vi "Load Words.vi"() -> (3 "Words":string[](array[string]))   [LabVIEW 2020]
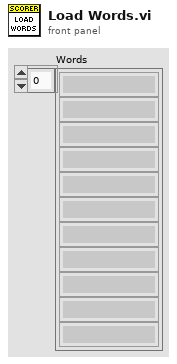
[diagram p1: front panel]
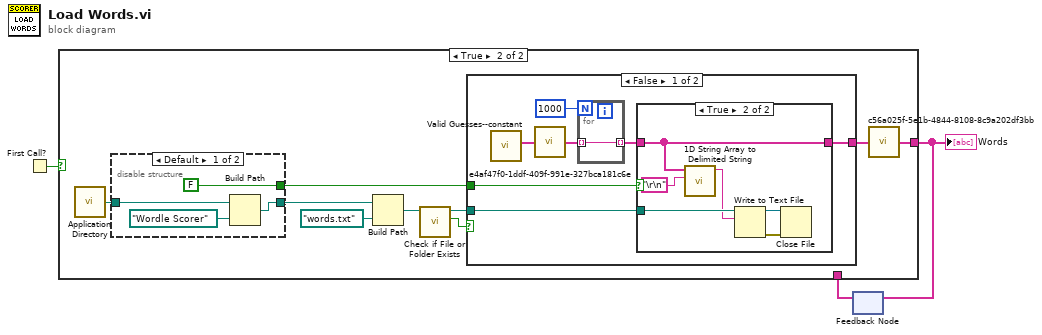
[diagram p0: block diagram]
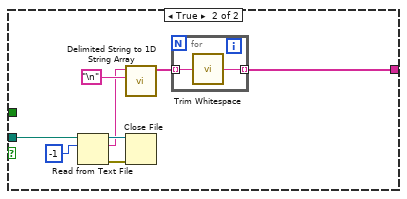
[diagram p4: hidden frame]
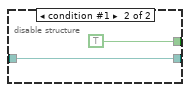
[diagram p5: hidden frame]
diagram:
  n1 = First Call?() -> (First Call?: T/F=w3:bool)
  n2 = feedback #1() -> (w2:string[])  [unwired: 1 in]
  n3 = case shown="True" w3 {
    tunnel: [w4 w5] -> w1
    tunnel: w2 -> [w4 _]
    frame False {
    }
    frame True {
      n4 = call <vilib>:"Application Directory.vi"() -> ("Application Directory"=w13:path)
      n5 = disable-structure shown="Default" {
        disable-tunnel: w13 -> [w42 w44]
        disable-tunnel: [w40 w44] -> w12
        disable-tunnel: [FALSE TRUE] -> w9
        frame condition #0 (active) {
          n6 = Build Path(base path=w42, name or relative path=path "Wordle Scorer") -> (appended path=w40:path)
        }
        frame condition #1 {
        }
      }
      n7 = Build Path(base path=w12, name or relative path=path "words.txt") -> (appended path=w10:path)
      n8 = call <vilib>:"Check if File or Folder Exists.vi"("path"=w10) -> ("file or folder exists?"=w8:bool, "dup path"=w7:path)  [unwired: 8 in, 1 out]
      n9 = case shown="False" w8 {
        tunnel: w9 -> [w20 _]
        tunnel: w7 -> [w19 w36]
        tunnel: [w14 w29] -> w6
        frame False {
          n10 = call "Valid Guesses--constant.vi"() -> ("Valid Guesses (array)"=w18:string[])  [unwired: 10 in, 1 out]
          n11 = call "e4af47f0-1ddf-409f-991e-327bca181c6e.vi"("array"=w18) -> ("shuffled array"=w16:string[])  [unwired: 4 in]
          n12 = for {
            N: 1000 -> [_]
            tunnel: w16 -> [w21] mode=indexing
            tunnel: [w21] -> w15 mode=indexing
          }
          n13 = case shown="True" w20 {
            tunnel: w19 -> [_ w27]
            tunnel: w15 -> [w22 w25]
            tunnel: [w22 w25] -> w14
            frame False {
            }
            frame True {
              n14 = call <vilib>:"1D String Array to Delimited String.vi"("delimiter"="\r\n", "string array"=w25) -> ("delimited string"=w26:string)  [unwired: 9 in]
              n15 = Write to Text File(file (use dialog)=w27, text=w26) -> (refnum out=w24:refnum<file>, error out=w23:errorcluster)  [unwired: 2 in, 1 out]
              n16 = Close File(refnum=w24, error in=w23) -> ()  [unwired: 2 out]
            }
          }
        }
        frame True {
          n17 = Read from Text File(file (use dialog)=w36, count=-1) -> (refnum out=w34:refnum<file>, text=w31:string, error out=w33:errorcluster)  [unwired: 2 in, 1 out]
          n18 = call <vilib>:"Delimited String to 1D String Array.vi"("delimiter"="\n", "delimited string"=w31) -> ("string array"=w30:string[])  [unwired: 9 in]
          n19 = Close File(refnum=w34, error in=w33) -> ()  [unwired: 2 out]
          n20 = for {
            tunnel: w30 -> [w38] mode=indexing
            tunnel: [w37] -> w29 mode=indexing
            n21 = call <vilib>:"Trim Whitespace.vi"("string"=w38) -> ("trimmed string"=w37:string)  [unwired: 1 in]
          }
        }
      }
      n22 = call "c56a025f-5e1b-4844-8108-8c9a202df3bb.vi"("array"=w6) -> ("shuffled array"=w5:string[])  [unwired: 4 in]
    }
  }
  "Words" <- w1
  n23 = feedback-in #1(w1) -> ()
